vi "checkValues.vi"(10 "Threshold":dbl=50.0 format="%#_13g", 11 "CheckData in":refnum<class "CheckData.lvclass">) -> (2 "Fault":bool, 3 "CheckData out":refnum<class "CheckData.lvclass">)   [LabVIEW 2017, in "CheckData.lvclass"]
uses:
  CheckData.lvclass
  CheckData.lvclass/CheckData.ctl
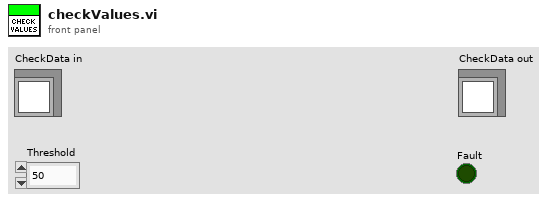
[diagram p1: front panel]
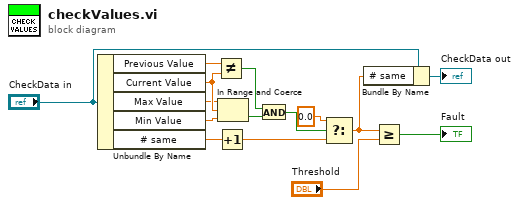
[diagram p0: block diagram]
diagram:
  n1 = Unbundle By Name("CheckData in") -> ("Previous Value"=w6:dbl, "Current Value"=w5:dbl, "Max Value"=w4:dbl, "Min Value"=w3:dbl, "# same"=w12:dbl)
  n2 = Not Equal?(x=w6, y=w5) -> (x != y?=w8:bool)
  n3 = Increment(x=w12) -> (x+1=w11:dbl)
  n4 = In Range and Coerce(upper limit=w4, x=w5, lower limit=w3) -> (In Range?=w7:bool)  [unwired: 1 out]
  n5 = And(x=w8, y=w7) -> (x .and. y?=w10:bool)
  n6 = Select(t=0.0, s=w10, f=w11) -> (s? t:f=w13:dbl)
  n7 = Bundle By Name(cluster="CheckData in", "# same"=w13) -> (→"CheckData out":refnum<class "CheckData.lvclass">)
  n8 = Greater Or Equal?(x=w13, y="Threshold") -> (x >= y?=→"Fault":bool)
